vi "addToImageStringQ.vi"(8 "error in (no error)":errorcluster, 10 "ImageString":string, 11 "ImageStreamDecoder in":refnum<class "ImageStreamDecoder.lvclass">) -> (0 "error out":errorcluster, 3 "ImageStreamDecoder out":refnum<class "ImageStreamDecoder.lvclass">)   [LabVIEW 2009, in "Hardware.lvlib" / "HWControllers.lvlib" / "ImageStreamDecoder.lvclass"]
uses:
  ImageStreamDecoder.lvclass
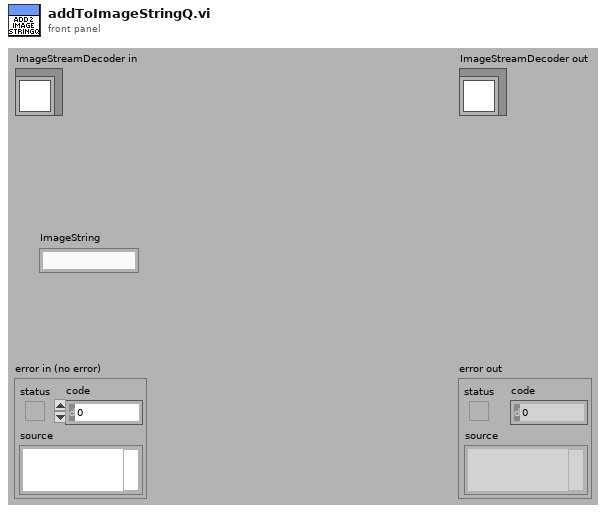
[diagram p1: front panel]
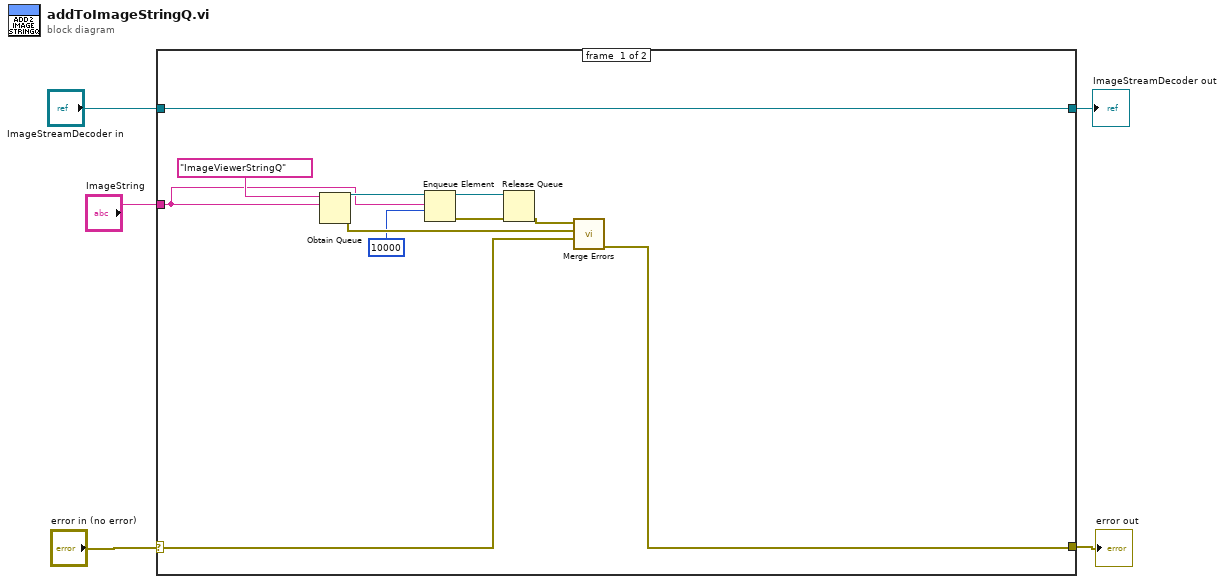
[diagram p0: block diagram]
diagram:
  n1 = case shown="No Error" "error in (no error)" {
    selector: "error in (no error)" -> [w9 w18]
    tunnel: [w8 w18] -> w4
    tunnel: [w16 w17] -> w2
    tunnel: "ImageStreamDecoder in" -> [w16 w17]
    tunnel: "ImageString" -> [w6 _]
    frame #0 {
      n2 = Obtain Queue(name (unnamed)="ImageViewerStringQ", element data type=w6) -> (queue out=w15:refnum<queue>, error out=w10:errorcluster)  [unwired: 3 in, 1 out]
      n3 = Enqueue Element(queue=w15, element=w6, timeout in ms (-1)=10000) -> (queue out=w13:refnum<queue>, error out=w14:errorcluster)  [unwired: 1 in, 1 out]
      n4 = Release Queue(queue=w13, error in (no error)=w14) -> (error out=w11:errorcluster)  [unwired: 1 in, 2 out]
      n5 = call <vilib>:"Merge Errors.vi"("error in 3 (no error)"=w9, "error in 2 (no error)"=w10, "error in 1 (no error)"=w11) -> ("error out"=w8:errorcluster)  [unwired: 4 in]
    }
    frame #1 {
    }
  }
  "error out" <- w4
  "ImageStreamDecoder out" <- w2
